vi "Interpolate1DArraySafe.vi"(10 "Fractional Index":dbl, 11 "Array":dbl[](array[numeric])) -> (3 "Numeric out":dbl)   [LabVIEW 2021]
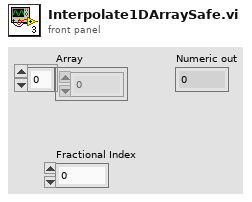
[diagram p1: front panel]
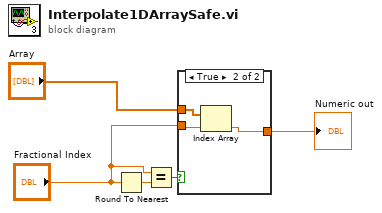
[diagram p0: block diagram]
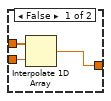
[diagram p2: hidden frame]
diagram:
  n1 = Round To Nearest(number="Fractional Index") -> (nearest integer value=w3:dbl)
  n2 = Equal?(x="Fractional Index", y=w3) -> (x = y?=w1:bool)
  n3 = case shown="True" w1 {
    tunnel: "Array" -> [w8 w11]
    tunnel: [w7 w9] -> w4
    tunnel: "Fractional Index" -> [w6 w10]
    frame False {
      n4 = Interpolate 1D Array(1:w6, 2:w8) -> (0:w7:dbl)
    }
    frame True {
      n5 = Index Array(array=w11, index=w10) -> (element=w9:dbl)
    }
  }
  "Numeric out" <- w4
